vi "CMDCreator.vi"(3 "Data":u8, 4 "DevCmd":T1 items=["WriteAddr"=81, "Enable"=80, "Red"=66, "Green"=65, "TurnOn"=49, "Shutdown"=48, "GetESD"=34], 5 "Addr":u8) -> (1 "Buff":string)   [LabVIEW 2012, in "DevControl.lvclass"]
uses:
  DevControl.lvclass
  DevCmd.ctl
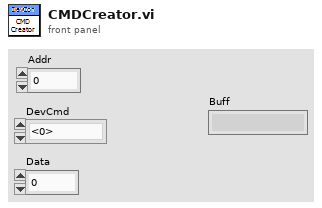
[diagram p1: front panel]
types:
  T1 = typedef "DevControl.lvclass/DevCmd.ctl" = u8
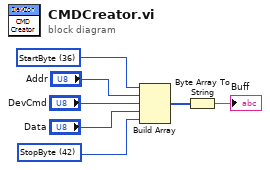
[diagram p0: block diagram]
diagram:
  w4 = u8 42 items=["StopByte"=42, "StartByte"=36] ("FunByte")
  w6 = u8 36 items=["StopByte"=42, "StartByte"=36] ("FunByte")
  n1 = Build Array(w6, "Addr", "DevCmd", "Data", w4) -> (w2:T1[])
  n2 = Byte Array To String(unsigned byte array=w2) -> (string=→"Buff":string)
